vi "sv_to_file_lfTester.vi"(1 "Test case":string(combo)="Power(W)", 2 "Illasco SN":string, 3 "Measured Value":dbl, 4 "Calculated voltage":dbl, 5 "Dataset divide 15":i32, 6 "Error in":errorcluster, 7 "Current(A) Input":dbl, 8 "Data file directory":path, 9 "Whether first line":bool, 10 "Start time":timestamp) -> (0 "Error out":errorcluster)   [LabVIEW 2017]
uses:
  <vilib>/Utility/file.llb/Write Delimited Spreadsheet (string).vi
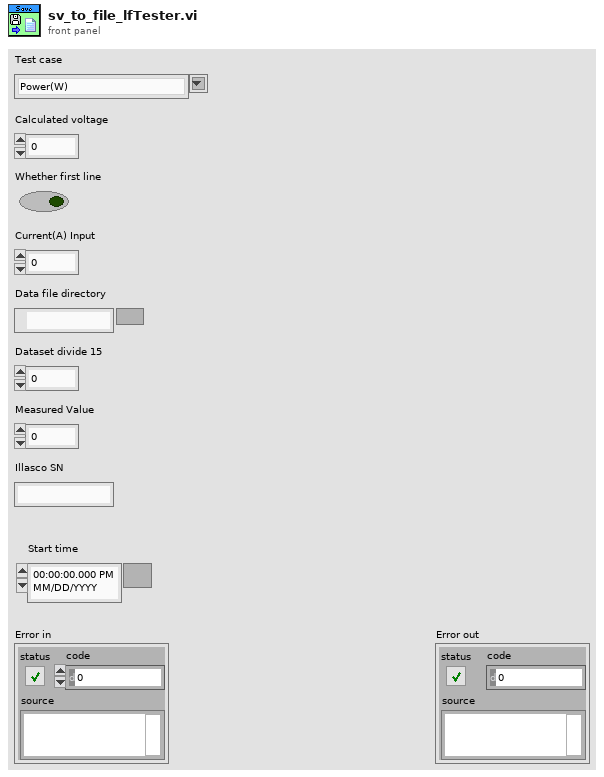
[diagram p1: front panel]
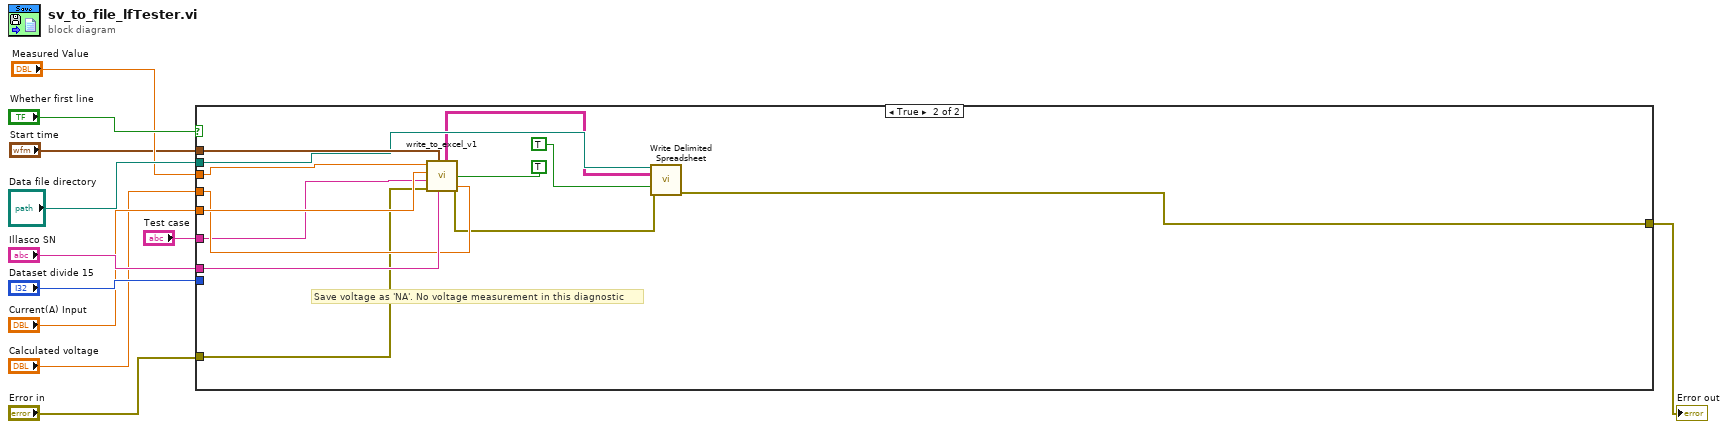
[diagram p0: block diagram]
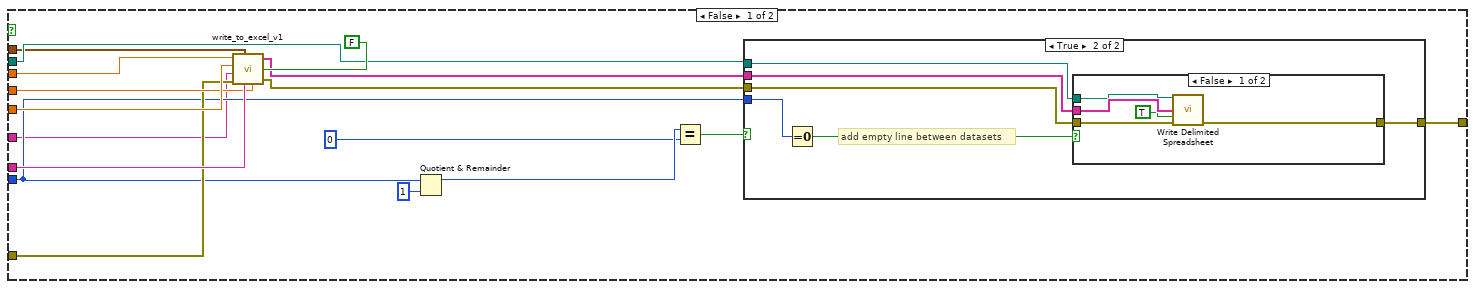
[diagram p2: hidden frame]
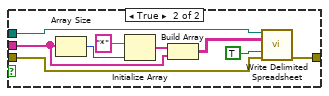
[diagram p4: hidden frame]
diagram:
  n1 = case shown="True" "Whether first line" {
    tunnel: "Measured Value" -> [w27 w62]
    tunnel: "Illasco SN" -> [w28 w61]
    tunnel: "Current(A) Input" -> [w26 w60]
    tunnel: "Calculated voltage" -> [w25 w59]
    tunnel: "Start time" -> [w19 w58]
    tunnel: "Data file directory" -> [w23 w56]
    tunnel: "Error in" -> [w22 w53]
    tunnel: [w20 w51] -> w3
    tunnel: "Dataset divide 15" -> [w13 _]
    tunnel: "Test case" -> [w12 w50]
    frame False {
      n2 = call "write_to_excel_v1.vi"("Voltage"=w25, "First(g), Other(k)"=FALSE, "Illasco SN"=w28, "error in (no error)"=w22, "Test case"=w12, "Execution Start"=w19, "Current"=w26, "Measured value"=w27) -> ("error out"=w21:errorcluster, "Array 1D"=w18:string[])  [unwired: 1 out]
      n3 = Quotient & Remainder(x=w13, y=1) -> (x-y*floor(x/y)=w16:i32)  [unwired: 1 out]
      n4 = Equal?(x=w16, y=0) -> (x = y?=w14:bool)
      n5 = case shown="True" w14 {
        tunnel: w23 -> [_ w35]
        tunnel: w21 -> [w29 w34]
        tunnel: [w29 w33] -> w20
        tunnel: w18 -> [_ w32]
        tunnel: w13 -> [_ w31]
        frame False {
        }
        frame True {
          # "add empty line between datasets"
          n6 = Equal To 0?(x=w31) -> (x = 0?=w30:bool)
          n7 = case shown="False" w30 {
            tunnel: w35 -> [w39 w49]
            tunnel: w34 -> [w37 w48]
            tunnel: [w36 w47] -> w33
            tunnel: w32 -> [w40 w41]
            frame False {
              n8 = call-poly <vilib>:"Write Delimited Spreadsheet.vi"("file path (dialog if empty)"=w39, "1D data"=w40, "append to file? (new file:F)"=TRUE, "error in (no error)"=w37) -> ("error out"=w36:errorcluster)  [unwired: 10 in, 1 out]
            }
            frame True {
              n9 = Array Size(array=w41) -> (size(s)=w45:i32)
              n10 = Initialize Array("*" ("element"), w45) -> (w42:string[])
              n11 = Build Array(w42, w41) -> (w44:string[][])
              n12 = call-poly <vilib>:"Write Delimited Spreadsheet.vi"("file path (dialog if empty)"=w49, "2D data"=w44, "append to file? (new file:F)"=TRUE, "error in (no error)"=w48) -> ("error out"=w47:errorcluster)  [unwired: 10 in, 1 out]
            }
          }
        }
      }
    }
    frame True {
      # "Save voltage as 'NA'. No voltage measurement in this diagnostic"
      n13 = call "write_to_excel_v1.vi"("Voltage"=w59, "First(g), Other(k)"=TRUE, "Illasco SN"=w61, "error in (no error)"=w53, "Test case"=w50, "Execution Start"=w58, "Current"=w60, "Measured value"=w62) -> ("error out"=w52:errorcluster, "Array 2D"=w55:string[][])  [unwired: 1 out]
      n14 = call-poly <vilib>:"Write Delimited Spreadsheet.vi"("file path (dialog if empty)"=w56, "2D data"=w55, "append to file? (new file:F)"=TRUE, "error in (no error)"=w52) -> ("error out"=w51:errorcluster)  [unwired: 10 in, 1 out]
    }
  }
  "Error out" <- w3
